vi "Start All.vi"(7 "options":T1, 8 "error in (no error)":errorcluster, 11 "Thread Manager in":refnum<class "Thread Manager.lvclass">) -> (0 "error out":errorcluster, 3 "Thread Manager out":refnum<class "Thread Manager.lvclass">)   [LabVIEW 2017, in "DSF Core.lvlib" / "Thread Manager.lvclass"]
uses:
  Thread Manager.lvclass
  Thread/DSF Thread Options.ctl
  Thread Manager.lvclass/Thread Manager.ctl
  Thread/Thread.lvclass
  DSF Core.lvlib
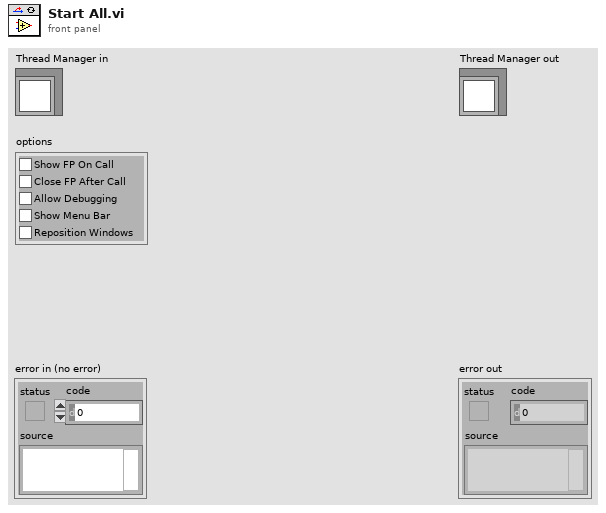
[diagram p1: front panel]
types:
  T1 = typedef "DSF Core.lvlib/DSF Thread Options.ctl" = cluster{"Show FP On Call":bool, "Close FP After Call":bool, "Allow Debugging":bool, "Show Menu Bar":bool, "Reposition Windows":bool}
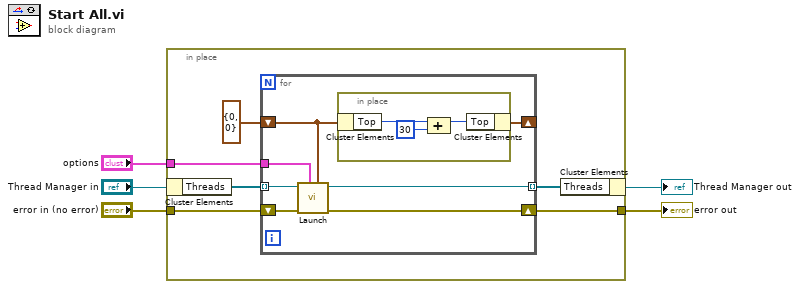
[diagram p0: block diagram]
diagram:
  n1 = in-place {
    in-place-border: [w9] -> w3
    in-place-border: "error in (no error)" -> [w8]
    in-place-border: "options" -> [w6]
    n2 = in-place-cluster #1("Thread Manager in") -> ("Threads"=w11:refnum<class "Thread.lvclass">[])
    n3 = for {
      tunnel: w11 -> [w18] mode=indexing
      tunnel: [w17] -> w10 mode=indexing
      shift-right: [w15] -> w9
      shift-left: w8 -> [w16]
      shift-right: [w13] -> _
      shift-left: cluster{"Left":i16, "Top":i16} {"Left"=0, "Top"=0} ("window position") -> [w14]
      tunnel: w6 -> [w12]
      n4 = call "Launch.vi"("window position"=w14, "options"=w12, "error in (no error)"=w16, "Thread in"=w18) -> ("error out"=w15:errorcluster, "Thread out"=w17:refnum<class "Thread.lvclass">)  [unwired: 6 in]
      n5 = in-place {
        n6 = in-place-cluster #2(w14) -> ("Top"=w21:i16)
        n7 = Compound Arithmetic op=ADD(w21, i16 30 ("y")) -> (w19:i16)
        n8 = in-place-cluster #2("Top"=w19) -> (w13:cluster{"Left":i16, "Top":i16})
      }
    }
    n9 = in-place-cluster #1("Threads"=w10) -> (→"Thread Manager out":refnum<class "Thread Manager.lvclass">)
  }
  "error out" <- w3
